vi "vision_fg.vi"(3 "Action":T1, 4 "Menu":T2) -> (0 "State Out":T1, 1 "Enabled?":bool)   [LabVIEW 2012]
uses:
  typedefs/fg_typedef.ctl
  typedefs/vision enable.ctl
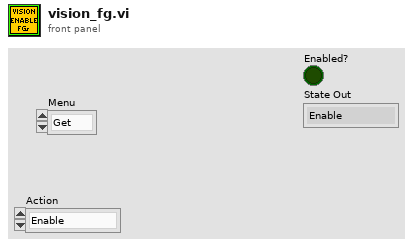
[diagram p1: front panel]
types:
  T1 = typedef "vision enable.ctl" = enum16{"Enable", "Disable", "Stop"}
  T2 = typedef "fg_typedef.ctl" = enum16{"Get", "Set"}
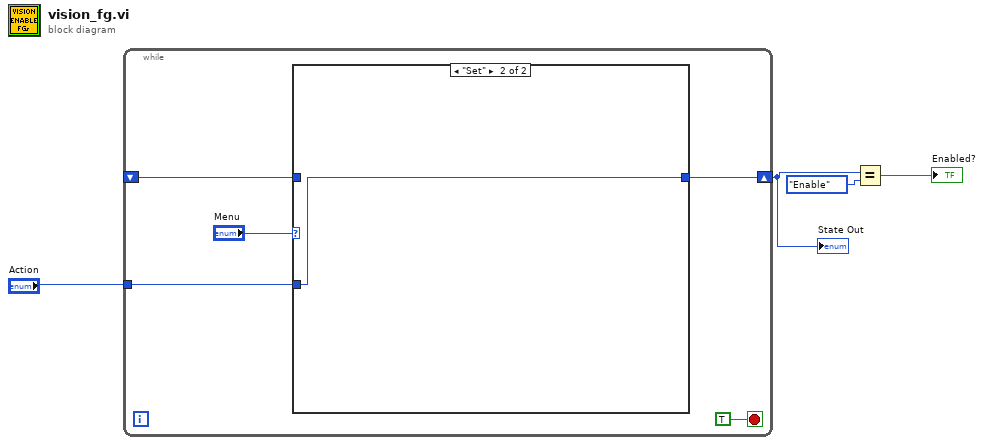
[diagram p0: block diagram]
diagram:
  n1 = while {
    shift-right: [w6] -> w3
    shift-left: _ -> [w7]
    tunnel: "Action" -> [w5]
    stop <- TRUE stop-if-true
    n2 = case shown="\"Set\"" "Menu" {
      tunnel: w7 -> [w10 _]
      tunnel: [w10 w11] -> w6
      tunnel: w5 -> [_ w11]
      frame "Get", Default {
      }
      frame "Set" {
      }
    }
  }
  "State Out" <- w3
  n3 = Equal?(x=w3, y=vision_enable."Enable") -> (x = y?=→"Enabled?":bool)
